vi "TDMS Upload Example.vi"() -> ()   [LabVIEW 2024]
doc: "TDMS upload example."
uses:
  Sift API/Sift Client.lvclass
panel:
  in  "Run Name":string="TDMS Upload Example"
  in  "Asset Name":string="LabVIEW-TDMS-Example"
  in  "Absolute Filepath":path
  out "Error":errorcluster
  in  "API Key":string
  in  "API URL":string
  # "Instructions\n\n1. Fill in the API URL and API Key. Visit this URL for more information on authentication\n    https://docs.siftstack.com/docs/api/authentication\n\n2. Select a TDMS file to upload. There is a \"sample_data.tdms\" file in the same Example directory of this VI.\n\n3. Run the VI.\n\n3. The VI should run to completetion with no errors. Navigate to the Sift home page and find the \n     Run to see the example data."
  # "Sift TDMS Upload Example"
  # "Run this example to test uploading TDMS files to Sift."
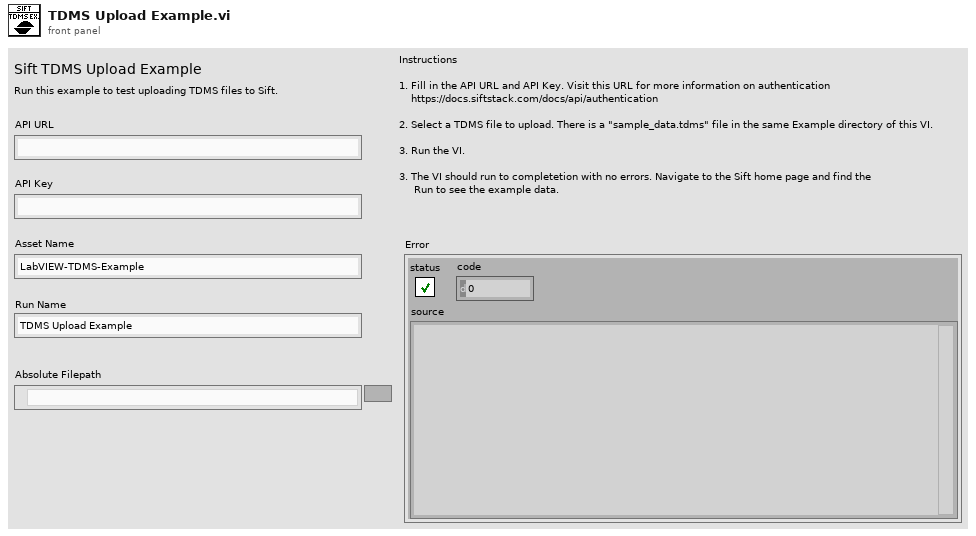
[diagram p1: front panel]
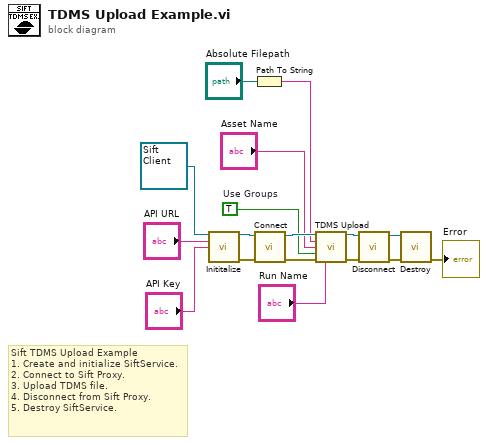
[diagram p0: block diagram]
diagram:
  w3 = TRUE  # Use Groups
  # "Sift TDMS Upload Example\n1. Create and initialize SiftService.\n2. Connect to Sift Proxy.\n3. Upload TDMS file.\n4. Disconnect from Sift Proxy.\n5. Destroy SiftService."
  n1 = call-dynamic "Inititalize.vi"("Sift Client in"=refnum<class "Sift Client.lvclass"> refnum ("Sift Client.lvlib:Sift Client.lvclass"), "API URL"="API URL", "API Key"="API Key") -> ("Sift Client out"=w13:refnum<class "Sift Client.lvclass">, "error out"=w12:errorcluster)  [unwired: 11 in]
  n2 = Path To String(path="Absolute Filepath") -> (string=w2:string)
  n3 = call-dynamic "Connect.vi"("error in (no error)"=w12, "Sift Client in"=w13) -> ("error out"=w10:errorcluster, "Sift Client out"=w11:refnum<class "Sift Client.lvclass">)  [unwired: 7 in, 1 out]
  n4 = call-dynamic "TDMS Upload.vi"("Sift Client in"=w11, "Filepath"=w2, "Asset Name"="Asset Name", "Group Into Components"=w3, "error in (no error)"=w10, "Run Name"="Run Name") -> ("Sift Client out"=w9:refnum<class "Sift Client.lvclass">, "error out"=w8:errorcluster)  [unwired: 8 in]
  n5 = call-dynamic "Disconnect.vi"("error in (no error)"=w8, "Sift Client in"=w9) -> ("error out"=w6:errorcluster, "Sift Client out"=w7:refnum<class "Sift Client.lvclass">)  [unwired: 8 in]
  n6 = call-dynamic "Destroy.vi"("error in (no error)"=w6, "Sift Client in"=w7) -> ("error out"=→"Error":errorcluster)  [unwired: 8 in, 1 out]
